vi "data-to-matlab.vi"(8 "error in (no error)":errorcluster, 11 "Config":T1 {"Hardware Configuration"."Sample mode" items=["Continuous Samples"=10123]}) -> (0 "error out":errorcluster)   [LabVIEW 2018]
uses:
  Settings/Settings.ctl
  Acquisition/Hardware Configuration.ctl
  Logging Configuration.ctl
  <vilib>/Waveform/WDTOps.llb/WDT Index Channel DBL.vi
  <vilib>/Waveform/WDTOps.llb/WDT Get Waveform Time Array DBL.vi
  Acquisition/Acquisition.lvlib
  Logging.lvlib
  Settings/Settings.lvlib
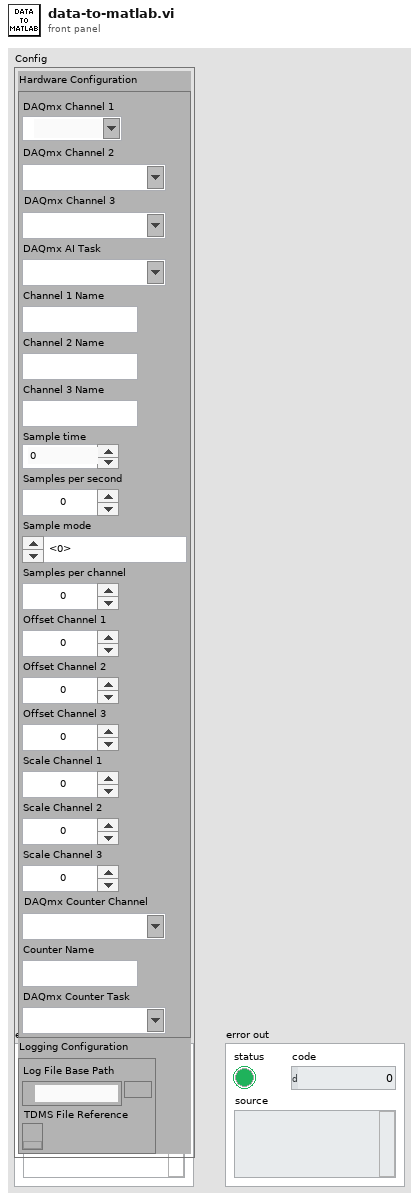
[diagram p1: front panel]
types:
  T1 = typedef "Settings.lvlib/Settings.ctl" = cluster{"Hardware Configuration":T2, "Logging Configuration":T3}
  T2 = typedef "Acquisition.lvlib/Hardware Configuration.ctl" = cluster{"DAQmx Channel 1":tag, "DAQmx Channel 2":tag, "DAQmx Channel 3":tag, "DAQmx AI Task":refnum<k21>, "Channel 1 Name":string, "Channel 2 Name":string, "Channel 3 Name":string, "Sample time":u32, "Samples per second":dbl, "Sample mode":u16, "Samples per channel":i32, "Offset Channel 1":dbl, "Offset Channel 2":dbl, "Offset Channel 3":dbl, "Scale Channel 1":dbl, "Scale Channel 2":dbl, "Scale Channel 3":dbl, "DAQmx Counter Channel":tag, "Counter Name":string, "DAQmx Counter Task":refnum<k21>}
  T3 = typedef "Logging.lvlib/Logging Configuration.ctl" = cluster{"Log File Base Path":path, "TDMS File Reference":refnum<k34>}
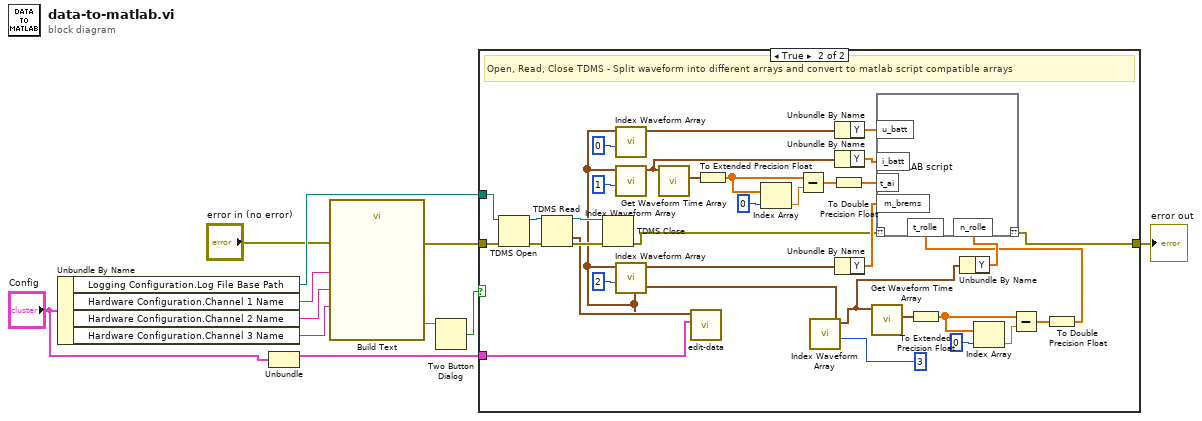
[diagram p0: block diagram]
diagram:
  n1 = Unbundle By Name("Config") -> ("Logging Configuration.Log File Base Path"=w9:path, "Hardware Configuration.Channel 1 Name"=w5:string, "Hardware Configuration.Channel 2 Name"=w6:string, "Hardware Configuration.Channel 3 Name"=w7:string)
  n2 = Unbundle("Config") -> ("Hardware Configuration"=w1:T2)  [unwired: 1 out]
  n3 = call "Build Text"("channel1"=w5, "channel2"=w6, "channel3"=w7, "error in (no error)"="error in (no error)") -> ("Result"=w4:string, "error out"=w11:errorcluster)  [unwired: 10 in]
  n4 = Two Button Dialog(message=w4) -> (T button?=w3:bool)  [unwired: 2 in]
  n5 = case shown="True" w3 {
    tunnel: w9 -> [_ w28]
    tunnel: [w12 w23] -> w10
    tunnel: w11 -> [w12 w27]
    tunnel: w1 -> [_ w25]
    frame False {
      # "If canceled, do nothing"
    }
    frame True {
      # "Open, Read, Close TDMS - Split waveform into different arrays and convert to matlab script compatible arrays"
      n6 = TDMS Open(8:w27, 11:w28) -> (0:w35:errorcluster, 3:w33:refnum<k34>)  [unwired: 5 in]
      n7 = TDMS Read(0:w33, 11:w35) -> (4:w34:refnum<k34>, 10:w26:waveform(dbl)[], 15:w36:errorcluster)  [unwired: 6 in, 3 out]
      n8 = TDMS Close(8:w36, 11:w34) -> (0:w24:errorcluster)  [unwired: 1 out]
      n9 = call "edit-data.vi"("Hardware Resources in"=w25, "data"=w26) -> ("Array of Waveform"=w22:waveform(dbl)[])  [unwired: 9 in]
      n10 = call-poly <vilib>:"Index Waveform Array.vi"("index"=0, "waveform array"=w22) -> ("waveform"=w38:waveform(dbl))  [unwired: 8 in, 1 out]
      n11 = call-poly <vilib>:"Index Waveform Array.vi"("index"=1, "waveform array"=w22) -> ("waveform"=w37:waveform(dbl))  [unwired: 8 in, 1 out]
      n12 = call-poly <vilib>:"Index Waveform Array.vi"("index"=2, "waveform array"=w22) -> ("waveform"=w44:waveform(dbl))  [unwired: 8 in, 1 out]
      n13 = call-poly <vilib>:"Get Waveform Time Array.vi"("waveform in"=w37) -> ("X array"=w40:timestamp[])  [unwired: 9 in, 1 out]
      n14 = To Extended Precision Float(1:w40) -> (0:w41:ext[])
      n15 = Index Array(array=w41, index=0) -> (element=w42:ext)
      n16 = Subtract(x=w41, y=w42) -> (x-y=w46:ext[])
      n17 = call-poly <vilib>:"Index Waveform Array.vi"("index"=3, "waveform array"=w22) -> ("waveform"=w15:waveform(dbl))  [unwired: 8 in, 1 out]
      n18 = To Double Precision Float(number=w46) -> (double precision float=w47:dbl[])
      n19 = Unbundle By Name(w38) -> ("Y"=w43:dbl[])
      n20 = Unbundle By Name(w37) -> ("Y"=w39:dbl[])
      n21 = Unbundle By Name(w44) -> ("Y"=w45:dbl[])
      n22 = call-poly <vilib>:"Get Waveform Time Array.vi"("waveform in"=w15) -> ("X array"=w17:timestamp[])  [unwired: 9 in, 1 out]
      n23 = To Extended Precision Float(1:w17) -> (0:w18:ext[])
      n24 = Unbundle By Name(w15) -> ("Y"=w14:dbl[])
      n25 = Index Array(array=w18, index=0) -> (element=w19:ext)
      n26 = Subtract(x=w18, y=w19) -> (x-y=w20:ext[])
      n27 = To Double Precision Float(number=w20) -> (double precision float=w13:dbl[])
      n28 = script code="MATLAB script"("??"=w24, "i_batt"=w39, "t_ai"=w47, "u_batt"=w43, "m_brems"=w45, "n_rolle"=w14, "t_rolle"=w13) -> ("??"=w23:errorcluster)
    }
  }
  "error out" <- w10
